vi "Stopped.vi"(6 "Teller":refnum<class "Teller.lvclass">, 9 "Error":errorcluster, 10 "Actor":refnum<class "Actor.lvclass">, 11 "Stopped in":refnum<class "Stopped.lvclass">) -> (0 "Error out":errorcluster, 3 "Stopped out":refnum<class "Stopped.lvclass">)   [LabVIEW 2025, in "jettl.lvlib" / "Stopped Msg.lvlib" / "Stopped.lvclass"]
uses:
  Stopped.lvclass
  Actor/Actor/Actor.lvclass
  Teller/Teller/Teller.lvclass
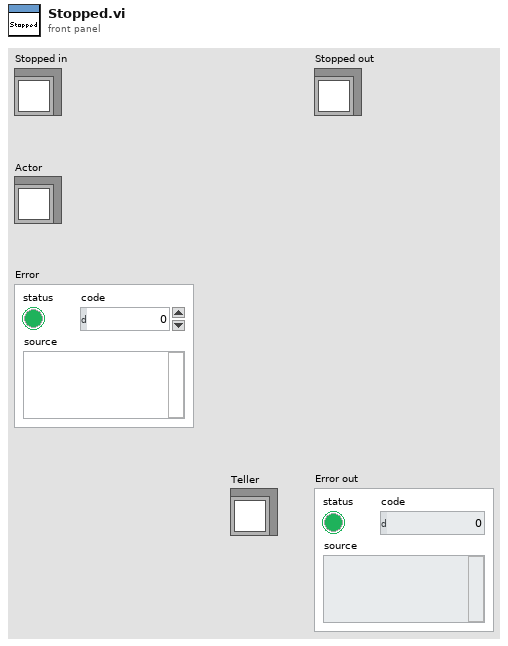
[diagram p1: front panel]
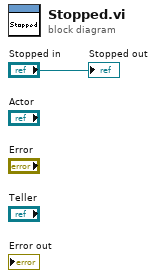
[diagram p0: block diagram]
diagram:
  "Stopped out" <- "Stopped in"
